vi "Delay Echo.vi"() -> ()   [LabVIEW 2014]
uses:
  <vilib>/eio/EIONode/EIONode.xnode
  <vilib>/rvi/eio/common/nirviEmuTemplateMethod_errors.vi
panel:
  in  "stop":bool
  in  "1/a":i16(knob) scale=2.0..20.0
  in  "Delay":i16(slide) scale=1.0..10.0
  in  "Count(Ticks)":u32(knob) caption="Ticks Sampling" scale=1.0..1000.0
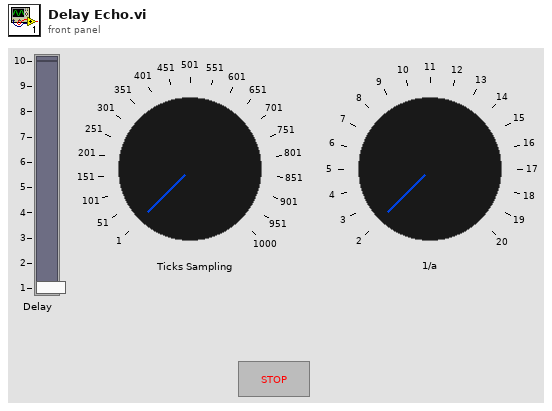
[diagram p1: front panel]
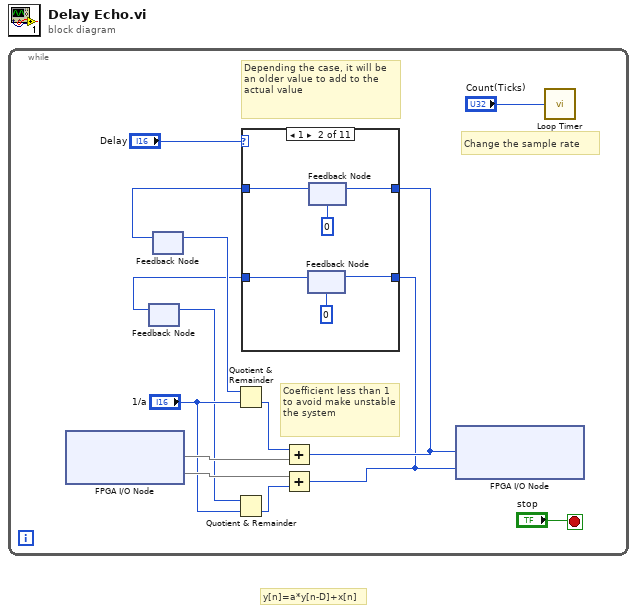
[diagram p0: block diagram]
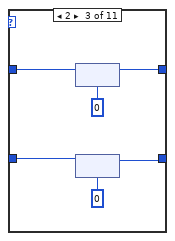
[diagram p3: hidden frame]
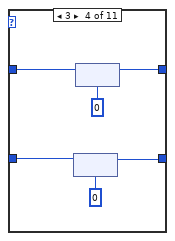
[diagram p4: hidden frame]
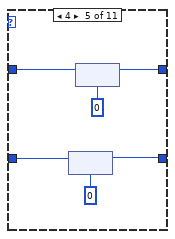
[diagram p5: hidden frame]
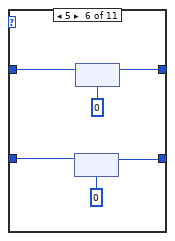
[diagram p6: hidden frame]
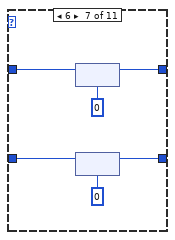
[diagram p7: hidden frame]
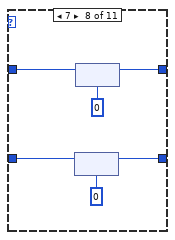
[diagram p8: hidden frame]
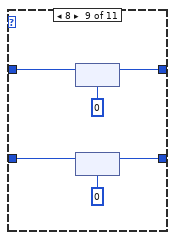
[diagram p9: hidden frame]
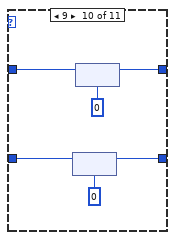
[diagram p10: hidden frame]
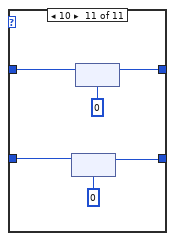
[diagram p11: hidden frame]
diagram:
  # "y[n]=a*y[n-D]+x[n]"
  n1 = while {
    stop <- "stop" stop-if-true
    # "Depending the case, it will be an older value to add to the actual value"
    # "Change the sample rate"
    # "Coefficient less than 1 to avoid make unstable the system"
    n2 = xnode "FPGA I/O Node"() -> ("AudioIn/Left"=w13, "AudioIn/Right"=w12)  [unwired: 2 in, 2 out]
    n3 = feedback #1() -> (w1:i16)  [unwired: 1 in]
    n4 = feedback #2() -> (w5:i16)  [unwired: 1 in]
    n5 = Quotient & Remainder(x=w5, y="1/a") -> (floor(x/y)=w11:i16)  [unwired: 1 out]
    n6 = Quotient & Remainder(x=w1, y="1/a") -> (floor(x/y)=w9:i16)  [unwired: 1 out]
    n7 = Add(x=w11, y=w13) -> (x+y=w7:i16)
    n8 = Add(x=w12, y=w9) -> (x+y=w3:i16)
    n9 = case shown="1" "Delay" {
      tunnel: w7 -> [w16 w22 w28 w34 w40 w46 w52 w58 w64 w70 w76]
      tunnel: [w16 w20 w26 w32 w38 w44 w50 w56 w62 w68 w74] -> w6
      tunnel: w3 -> [w15 w17 w23 w29 w35 w41 w47 w53 w59 w65 w71]
      tunnel: [w15 w18 w24 w30 w36 w42 w48 w54 w60 w66 w72] -> w2
      frame 0, Default {
      }
      frame 1 {
        n10 = feedback #3(i16 0) -> (w18:i16)
        n11 = feedback-in #3(w17) -> ()
        n12 = feedback #4(i16 0) -> (w20:i16)
        n13 = feedback-in #4(w22) -> ()
      }
      frame 2 {
        n14 = feedback #5(i16 0) -> (w26:i16)
        n15 = feedback-in #5(w28) -> ()
        n16 = feedback #6(i16 0) -> (w24:i16)
        n17 = feedback-in #6(w23) -> ()
      }
      frame 3 {
        n18 = feedback #7(i16 0) -> (w30:i16)
        n19 = feedback-in #7(w29) -> ()
        n20 = feedback #8(i16 0) -> (w32:i16)
        n21 = feedback-in #8(w34) -> ()
      }
      frame 4 {
        n22 = feedback #9(i16 0) -> (w36:i16)
        n23 = feedback-in #9(w35) -> ()
        n24 = feedback #10(i16 0) -> (w38:i16)
        n25 = feedback-in #10(w40) -> ()
      }
      frame 5 {
        n26 = feedback #11(i16 0) -> (w42:i16)
        n27 = feedback-in #11(w41) -> ()
        n28 = feedback #12(i16 0) -> (w44:i16)
        n29 = feedback-in #12(w46) -> ()
      }
      frame 6 {
        n30 = feedback #13(i16 0) -> (w50:i16)
        n31 = feedback-in #13(w52) -> ()
        n32 = feedback #14(i16 0) -> (w48:i16)
        n33 = feedback-in #14(w47) -> ()
      }
      frame 7 {
        n34 = feedback #15(i16 0) -> (w54:i16)
        n35 = feedback-in #15(w53) -> ()
        n36 = feedback #16(i16 0) -> (w56:i16)
        n37 = feedback-in #16(w58) -> ()
      }
      frame 8 {
        n38 = feedback #17(i16 0) -> (w62:i16)
        n39 = feedback-in #17(w64) -> ()
        n40 = feedback #18(i16 0) -> (w60:i16)
        n41 = feedback-in #18(w59) -> ()
      }
      frame 9 {
        n42 = feedback #19(i16 0) -> (w66:i16)
        n43 = feedback-in #19(w65) -> ()
        n44 = feedback #20(i16 0) -> (w68:i16)
        n45 = feedback-in #20(w70) -> ()
      }
      frame 10 {
        n46 = feedback #21(i16 0) -> (w72:i16)
        n47 = feedback-in #21(w71) -> ()
        n48 = feedback #22(i16 0) -> (w74:i16)
        n49 = feedback-in #22(w76) -> ()
      }
    }
    n50 = feedback-in #1(w2) -> ()
    n51 = feedback-in #2(w6) -> ()
    n52 = xnode "FPGA I/O Node"("AudioOut/Left"=w7, "AudioOut/Right"=w3) -> ()  [unwired: 2 in, 2 out]
    n53 = call "Loop Timer"("Count(Ticks)"="Count(Ticks)") -> ()  [unwired: 1 out]
  }
